vi "initiate.vi"(0 "reference in":refnum<class "GUI Controller.lvclass">, 5 "error in (no error)":errorcluster) -> (14 "reference out":refnum<class "GUI Controller.lvclass">, 19 "error out":errorcluster)   [LabVIEW 2015, in "GUI Controller.lvclass"]
uses:
  GUI Controller.lvclass
  Project Panels_class/Project Panels.lvclass
  SYS/File Controller_llb/File Controller.lvclass
  SYS/Subject Controller_llb/Subject Controller.lvclass
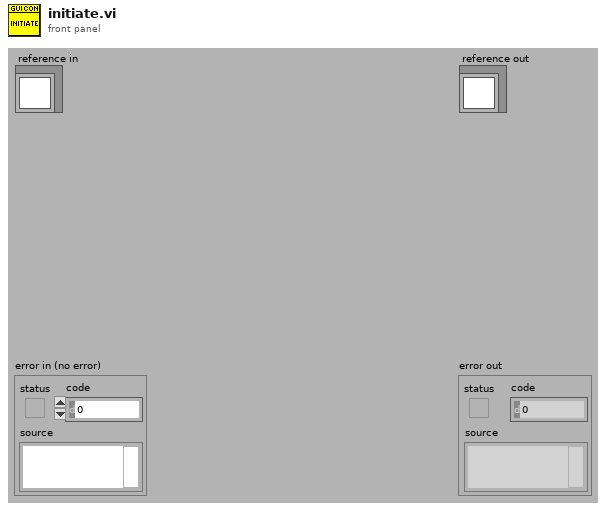
[diagram p1: front panel]
types:
  T1 = typedef "GUI Controller.lvclass/ObjectAttributesRef.ctl" = refnum<data-value>
  T2 = typedef "GUI Controller.lvclass/ObjectAttributes.ctl" = cluster{"MyAttribute":dbl, "state":T3, "project_panels_ref":refnum<class "Project Panels.lvclass">, "file_controller_ref":refnum<class "File Controller.lvclass">, "subject_controller_ref":refnum<class "Subject Controller.lvclass">}
  T3 = typedef "GUI Controller.lvclass/state.ctl" = enum16{"initiate", "AddNewFile", "ElaborateData", "CheckData", "waitEvent", "checkSubject", "ChangeSubject", "stop"}
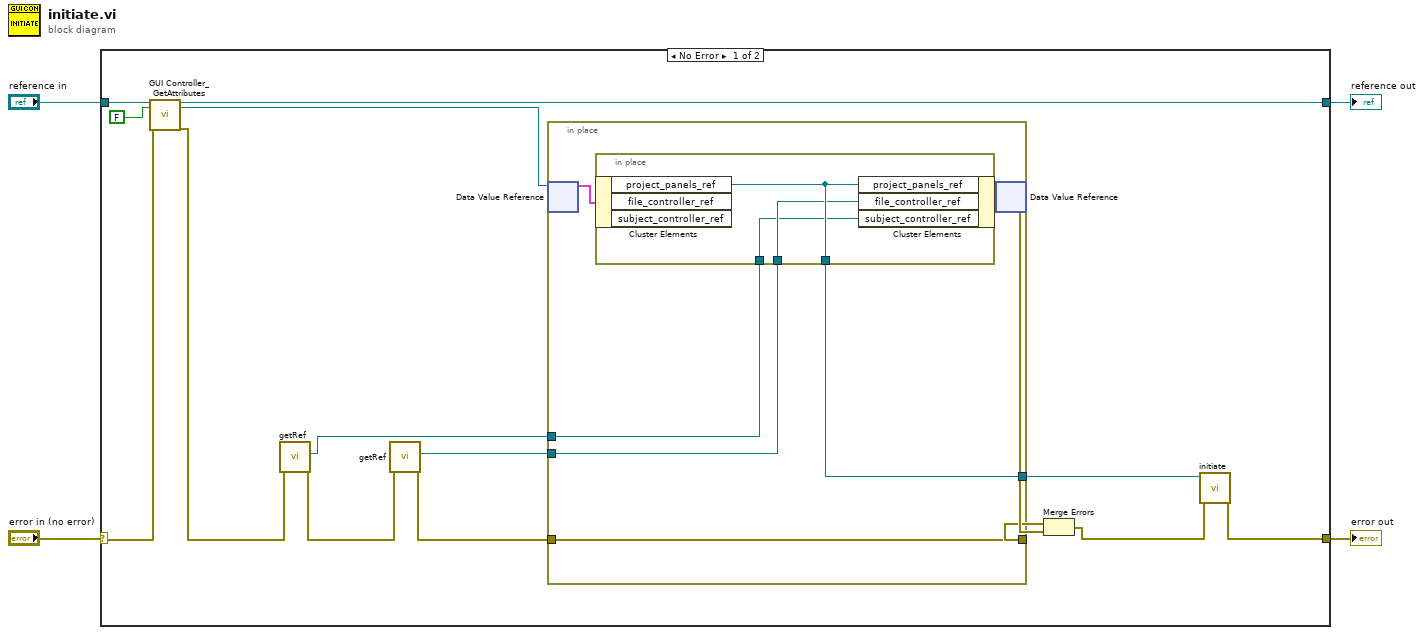
[diagram p0: block diagram]
diagram:
  n1 = case shown="No Error" "error in (no error)" {
    selector: "error in (no error)" -> [w15 w30]
    tunnel: [w10 w30] -> w3
    tunnel: [w14 w29] -> w1
    tunnel: "reference in" -> [w17 w29]
    frame No Error {
      n2 = call "GUI Controller_GetAttributes.vi"("reference in"=w17, "return data? (T)"=FALSE, "error in (no error)"=w15) -> ("reference out"=w14:refnum<class "GUI Controller.lvclass">, "attributes ref"=w13:T1, "error out"=w7:errorcluster)  [unwired: 13 in, 1 out]
      n3 = call "getRef.vi"("error in (no error)"=w7) -> ("error out"=w6:errorcluster, "subject_controller_ref"=w5:refnum<class "Subject Controller.lvclass">)  [unwired: 9 in]
      n4 = call "getRef.vi"("error in (no error)"=w6) -> ("error out"=w9:errorcluster, "File Controller.lvclass"=w8:refnum<class "File Controller.lvclass">)  [unwired: 9 in]
      n5 = in-place {
        in-place-border: w9 -> [w23]
        in-place-border: [w23] -> w18
        in-place-border: [w22] -> w12
        in-place-border: w8 -> [w21]
        in-place-border: w5 -> [w20]
        n6 = in-place-dvr #1(w13) -> (w24:T2)  [unwired: 1 out]
        n7 = in-place {
          in-place-border: [w28] -> w22
          in-place-border: w21 -> [w27]
          in-place-border: w20 -> [w26]
          n8 = in-place-cluster #2(w24) -> ("project_panels_ref"=w28:refnum<class "Project Panels.lvclass">)  [unwired: 2 out]
          n9 = in-place-cluster #2("project_panels_ref"=w28, "file_controller_ref"=w27, "subject_controller_ref"=w26) -> (w25:T2)
        }
        n10 = in-place-dvr #1(w25) -> (w19:errorcluster)  [unwired: 1 out]
      }
      n11 = Merge Errors(w18, w19) -> (w11:errorcluster)
      n12 = call "initiate.vi"("error in (no error)"=w11, "reference in"=w12) -> ("error out"=w10:errorcluster)  [unwired: 8 in, 1 out]
    }
    frame Error {
    }
  }
  "error out" <- w3
  "reference out" <- w1
